vi "Decode Binary Stream.vi"(11 "Bit Stream":bool[](array[boolean])) -> (2 "Packets Out":T1[](array[typedef]), 3 "Bit Stream Out":bool[](array[boolean]))   [LabVIEW 2019, in "Day 16.lvlib"]
uses:
  Day 16.lvlib
  Controls/Packet.ctl
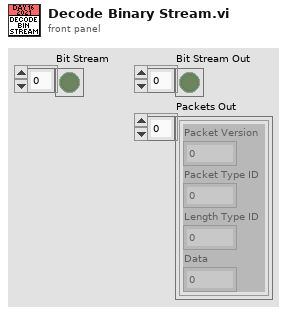
[diagram p1: front panel]
types:
  T1 = typedef "Day 16.lvlib/Packet.ctl" = cluster{"Packet Version":u32, "Packet Type ID":u32, "Length Type ID":u32, "Data":u64}
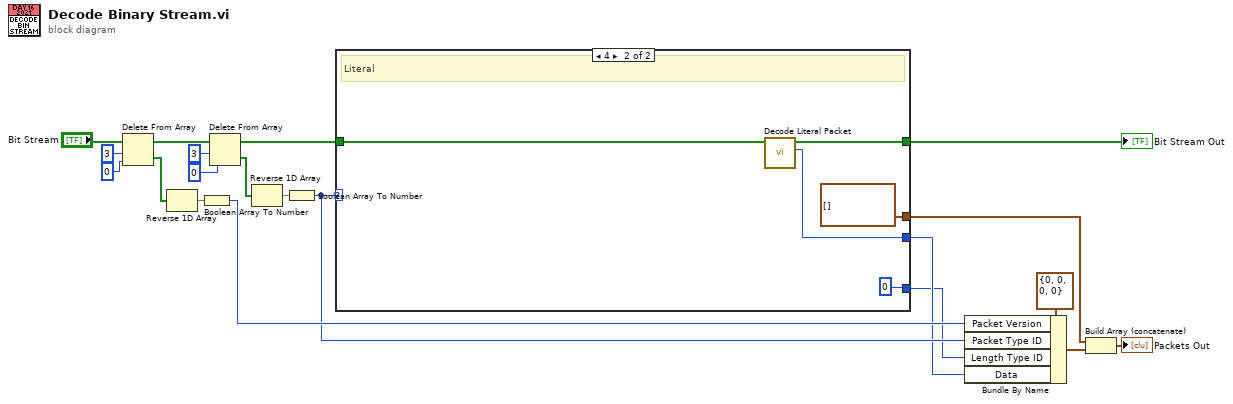
[diagram p0: block diagram]
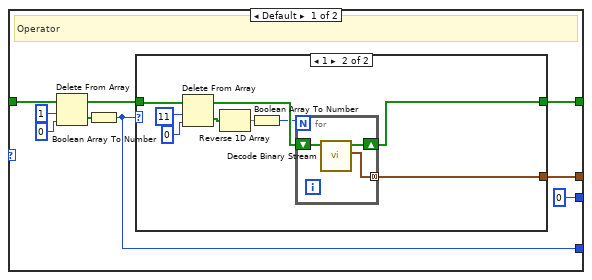
[diagram p2: hidden frame]
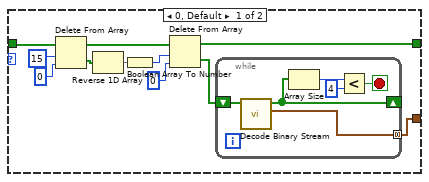
[diagram p3: hidden frame]
diagram:
  n1 = Delete From Array(array="Bit Stream", length=3, index=0) -> (deleted portion=w15:bool[], array with subset deleted=w17:bool[])
  n2 = Reverse 1D Array(array=w15) -> (reversed array=w14:bool[])
  n3 = Boolean Array To Number(Boolean array=w14) -> (number=w10:u32)
  n4 = Delete From Array(array=w17, length=3, index=0) -> (deleted portion=w12:bool[], array with subset deleted=w7:bool[])
  n5 = Reverse 1D Array(array=w12) -> (reversed array=w13:bool[])
  n6 = Boolean Array To Number(Boolean array=w13) -> (number=w9:u32)
  n7 = case shown="4" w9 {
    tunnel: w7 -> [w27 w63]
    tunnel: [w22 w60] -> w2
    tunnel: [u32 0 ("Data") w62] -> w6
    tunnel: [w24 u32 0 ("Length Type ID")] -> w5
    tunnel: [w21 T1[] [] ("Packets Out")] -> w1
    frame Default {
      # "Operator"
      n8 = Delete From Array(array=w27, length=1, index=0) -> (deleted portion=w26:bool[], array with subset deleted=w23:bool[])
      n9 = Boolean Array To Number(Boolean array=w26) -> (number=w24:u32)
      n10 = case shown="1" w24 {
        tunnel: w23 -> [w38 w53]
        tunnel: [w32 w47] -> w22
        tunnel: [w30 w50] -> w21
        frame 0, Default {
          n11 = Delete From Array(array=w38, length=15, index=0) -> (deleted portion=w35:bool[], array with subset deleted=w33:bool[])
          n12 = Reverse 1D Array(array=w35) -> (reversed array=w36:bool[])
          n13 = Boolean Array To Number(Boolean array=w36) -> (number=w34:u32)
          n14 = Delete From Array(array=w33, length=w34, index=0) -> (deleted portion=w31:bool[], array with subset deleted=w32:bool[])
          n15 = while {
            tunnel: [w45] -> w30 mode=concatenating
            shift-right: [w41] -> _
            shift-left: w31 -> [w46]
            stop <- w42 stop-if-true
            n16 = call "Decode Binary Stream.vi"("Bit Stream"=w46) -> ("Packets Out"=w45:T1[], "Bit Stream Out"=w41:bool[])  [unwired: 9 in]
            n17 = Array Size(array=w41) -> (size(s)=w44:i32)
            n18 = Less?(x=w44, y=4) -> (x < y?=w42:bool)
          }
        }
        frame 1 {
          n19 = Delete From Array(array=w53, length=11, index=0) -> (deleted portion=w51:bool[], array with subset deleted=w49:bool[])
          n20 = Reverse 1D Array(array=w51) -> (reversed array=w52:bool[])
          n21 = Boolean Array To Number(Boolean array=w52) -> (number=w48:u32)
          n22 = for {
            N: w48 -> [_]
            tunnel: [w57] -> w50 mode=concatenating
            shift-right: [w56] -> w47
            shift-left: w49 -> [w58]
            n23 = call "Decode Binary Stream.vi"("Bit Stream"=w58) -> ("Packets Out"=w57:T1[], "Bit Stream Out"=w56:bool[])  [unwired: 9 in]
          }
        }
      }
    }
    frame 4 {
      # "Literal"
      n24 = call "Decode Literal Packet.vi"("Bit Stream In"=w63) -> ("Data"=w62:u64, "Bit Stream Out"=w60:bool[])  [unwired: 9 in]
    }
  }
  "Bit Stream Out" <- w2
  n25 = Bundle By Name(cluster=T1 {"Packet Version"=0, "Packet Type ID"=0, "Length Type ID"=0, "Data"=0} ("Packet"), "Packet Version"=w10, "Packet Type ID"=w9, "Length Type ID"=w5, "Data"=w6) -> (w8:T1)
  n26 = Build Array (concatenate)(w1, w8) -> (→"Packets Out":T1[])
